vi "SUB_Get Window Handle.vi"(3 "Window Name":string) -> (1 "Window Handle":i32)   [LabVIEW 2015]
uses:
  user32.dll
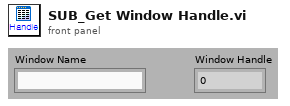
[diagram p1: front panel]
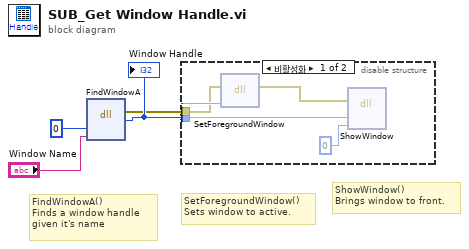
[diagram p0: block diagram]
diagram:
  # "ShowWindow()\nBrings window to front."
  # "SetForegroundWindow()\nSets window to active."
  # "FindWindowA()\nFinds a window handle \ngiven it's name"
  n1 = dll-call lib="user32.dll" fn="FindWindowA"("arg1"=0, "arg2"="Window Name") -> (error out=w1:errorcluster, "return type"=w2:i32)  [unwired: 4 in, 2 out]
  "Window Handle" <- w2
  n2 = disable-structure shown="비활성화" {
    disable-tunnel: w2 -> [w7 _]
    disable-tunnel: w1 -> [w6 _]
    frame Disabled {
      n3 = dll-call lib="user32.dll" fn="SetForegroundWindow"(error in=w6, "arg1"=w7) -> (error out=w5:errorcluster)  [unwired: 3 in, 2 out]
      n4 = dll-call lib="user32.dll" fn="ShowWindow"(error in=w5, "arg1"=w7, "arg2"=0) -> ()  [unwired: 4 in, 3 out]
    }
    frame Enabled {
    }
  }
